vi "Log Error.vi"(8 "error in (no error)":errorcluster, 10 "Error Data":T1, 11 "Car Wash Controller in":refnum<class "Car Wash Controller.lvclass">) -> (0 "error out":errorcluster, 3 "Car Wash Controller out":refnum<class "Car Wash Controller.lvclass">)   [LabVIEW 2019, in "Car Wash Controller.lvlib" / "Car Wash Controller.lvclass"]
uses:
  Car Wash Controller.lvclass
  Error Level.ctl
  States -Enum.ctl
  Wash Steps.ctl
  Error Data.ctl
panel:
  # "EH2A\nEH2B\nEH2C\nEH2D"
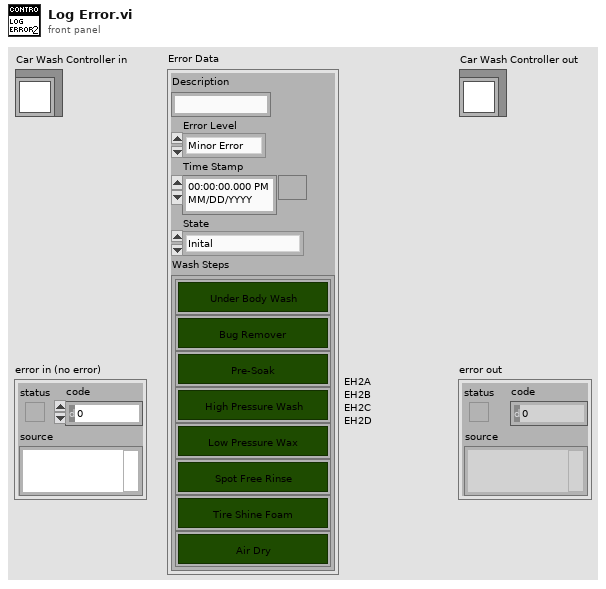
[diagram p1: front panel]
types:
  T1 = typedef "Car Wash Controller.lvlib/Car Wash Controller.lvclass/Error Data.ctl" = cluster{"Description":string, "Error Level":T2, "Time Stamp":timestamp, "State":T3, "Wash Steps":T4}
  T2 = typedef "Car Wash Controller.lvlib/Car Wash Controller.lvclass/Error Level.ctl" = enum16{"Minor Error", "Wash Cycle Error", "System Error"}
  T3 = typedef "Car Wash Controller.lvlib/Car Wash Controller.lvclass/States -Enum.ctl" = enum16{"Inital", "Wait for Start", "Start", "Wait for Vehicle Position", "Wash Step Execution", "Wash Step/Cycle Completion", "Wash Exit", "Wash Abort/Terminate State"}
  T4 = typedef "Car Wash Controller.lvlib/Car Wash Controller.lvclass/Wash Steps.ctl" = cluster{"Under Body Wash":bool, "Bug Remover":bool, "Pre-Soak":bool, "High Pressure Wash (Default)":bool, "Low Pressure Wax":bool, "Spot Free Rinse":bool, "Tire Shine Foam":bool, "Air Dry":bool}
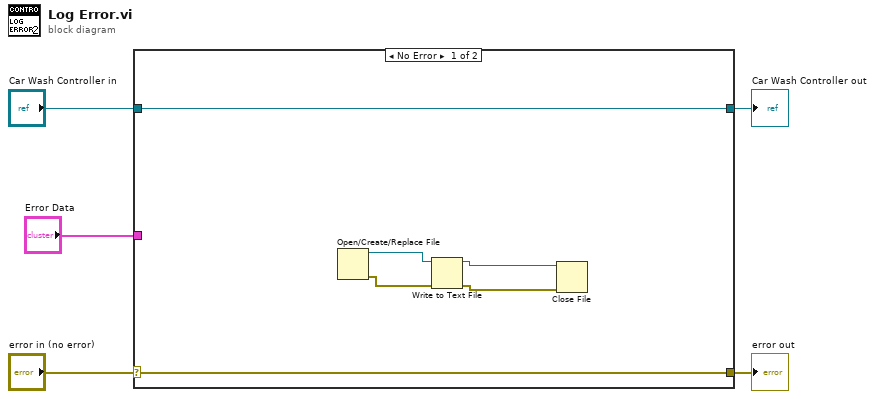
[diagram p0: block diagram]
diagram:
  n1 = case shown="No Error" "error in (no error)" {
    selector: "error in (no error)" -> [w10 w13]
    tunnel: [w10 w13] -> w4
    tunnel: [w11 w12] -> w2
    tunnel: "Car Wash Controller in" -> [w11 w12]
    tunnel: "Error Data" -> [_ _]
    frame No Error {
      n2 = Open/Create/Replace File() -> (refnum out=w9:refnum<file>, error out=w7:errorcluster)  [unwired: 6 in, 1 out]
      n3 = Write to Text File(file (use dialog)=w9, error in=w7) -> (refnum out=w8:refnum<file>, error out=w6:errorcluster)  [unwired: 2 in, 1 out]
      n4 = Close File(refnum=w8, error in=w6) -> ()  [unwired: 2 out]
    }
    frame Error {
    }
  }
  "error out" <- w4
  "Car Wash Controller out" <- w2
